vi "Configure Edge Trigger.vi"(0 "RedPitaya connection in":refnum<k5>, 1 "Trigger Delay mode":string(combo), 2 "Delay (ns)":i32 max=16348, 3 "Delay (# Samples)":i32 max=16348, 4 "Trigger Level (0 mV)":i32=-21000, 5 "error in":errorcluster, 12 "timeout ms (2000)":i32=2000) -> (14 "RedPitaya connection out":refnum<k5>, 19 "error out":errorcluster)   [LabVIEW 2010, in "RedPitaya.lvlib"]
doc: "Configures edge trigger settings. An edge trigger occurs when the trigger signal passes through the voltage threshold that you specify with the <B>Trigger Level</B> control.\n\nTo set acquisition trigger delay first select units in which you want to set by input <b>Trigger Delay mode</b>."
uses:
  RedPitaya.lvlib
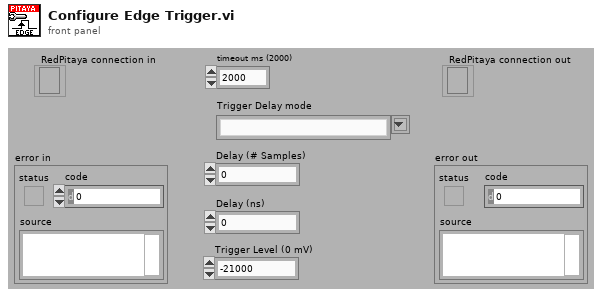
[diagram p1: front panel]
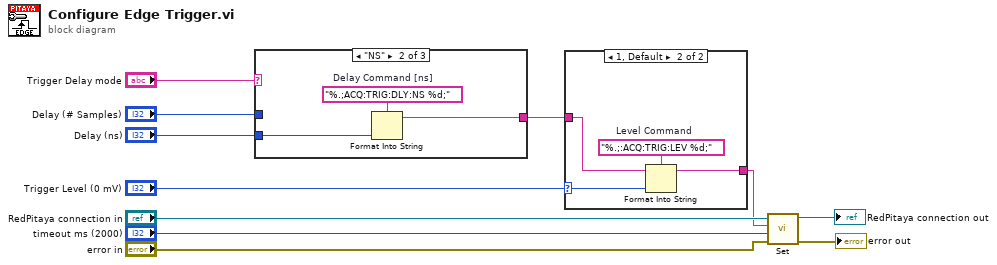
[diagram p0: block diagram]
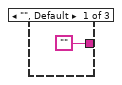
[diagram p3: hidden frame]
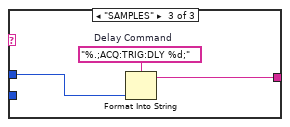
[diagram p4: hidden frame]
diagram:
  n1 = case shown="\"NS\"" "Trigger Delay mode" {
    tunnel: ["" w14 w17] -> w8
    tunnel: "Delay (ns)" -> [_ w13 _]
    tunnel: "Delay (# Samples)" -> [_ _ w16]
    frame "", Default {
    }
    frame "NS" {
      w15 = "%.;ACQ:TRIG:DLY:NS %d;"  # Delay Command [ns]
      n2 = Format Into String(format string=w15, w13) -> (resulting string=w14:string)  [unwired: 2 in, 1 out]
    }
    frame "SAMPLES" {
      w18 = "%.;ACQ:TRIG:DLY %d;"  # Delay Command
      n3 = Format Into String(format string=w18, w16) -> (resulting string=w17:string)  [unwired: 2 in, 1 out]
    }
  }
  n4 = case shown="1, Default" "Trigger Level (0 mV)" {
    selector: "Trigger Level (0 mV)" -> [_ w20]
    tunnel: w8 -> [w19 w22]
    tunnel: [w19 w21] -> w3
    frame -21000 {
    }
    frame 1, Default {
      w23 = "%.;:ACQ:TRIG:LEV %d;"  # Level Command
      n5 = Format Into String(format string=w23, initial string=w22, w20) -> (resulting string=w21:string)  [unwired: 1 in, 1 out]
    }
  }
  n6 = call "Set.vi"("error in"="error in", "timeout ms (2000)"="timeout ms (2000)", "SCPI Message"=w3, "RedPitaya connection in"="RedPitaya connection in") -> ("error out"=→"error out":errorcluster, "RedPitaya connection out"=→"RedPitaya connection out":refnum<k5>)  [unwired: 5 in, 1 out]
